vi "Untitled 12.vi"() -> ()   [LabVIEW 2011]
uses:
  james/LabView/AOD_Control/SerialController/Serial Controller.lvclass
  <vilib>/Instr/_visa.llb/VISA Configure Serial Port (Instr).vi
  <vilib>/Instr/_visa.llb/VISA Set IO Buffer Mask.ctl
panel:
  in  "VISA resource name":refnum<visa-resource-name>="COM2"
  in  "baud rate (9600)":u32=9600
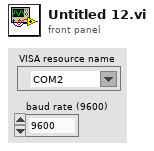
[diagram p1: front panel]
types:
  T1 = typedef "VISA Set IO Buffer Mask.ctl" = u16
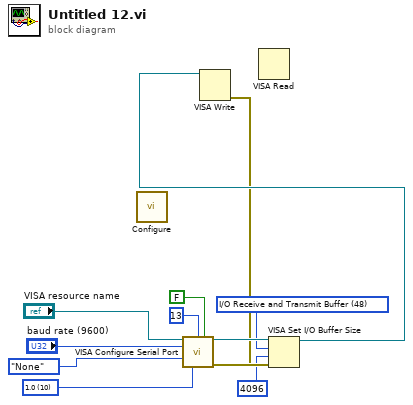
[diagram p0: block diagram]
diagram:
  w9 = T1 48 items=["I/O Receive Buffer"=16, "I/O Transmit Buffer"=32, "I/O Receive and Transmit Buffer"=48] ("Mask")
  w8 = u16 10 items=["1.0"=10, "1.5"=15, "2.0"=20] ("stop bits (10: 1 bit)")
  n1 = call-dynamic "Configure.vi"() -> ()  [unwired: 10 in, 2 out]
  n2 = call-poly "VISA Configure Serial Port"("VISA resource name"="VISA resource name", "termination char\n(0xA = '\\n' = LF)"=u8 13 ("termination char\n(0xA = '\\n' = LF)"), "Enable Termination\nChar (T)"=FALSE ("Enable Termination\nChar (T)"), "baud rate (9600)"="baud rate (9600)", "parity (0:none)"=enum16{"None", "Odd", "Even", "Mark", "Space"}."None", "stop bits (10: 1 bit)"=w8) -> ("VISA resource name out"=w11:refnum<visa-resource-name>, "error out"=w12:errorcluster)  [unwired: 8 in]
  n3 = VISA Read() -> ()  [unwired: 3 in, 4 out]
  n4 = VISA Set I/O Buffer Size(VISA resource name=w11, mask (16)=w9, size (4096)=u32 4096, error in (no error)=w12) -> (VISA resource name out=w2:refnum<visa-resource-name>, error out=w1:errorcluster)
  n5 = VISA Write(VISA resource name=w2, error in (no error)=w1) -> ()  [unwired: 1 in, 3 out]
